vi "2DdblArrayTostrTable.vi"(7 "RowsAreStrings (f)":bool, 11 "dbl2DArray":dbl[][](array[numeric])) -> (3 "strTable":string[][](table))   [LabVIEW 2014, in "Framework.lvlib"]
uses:
  Framework.lvlib
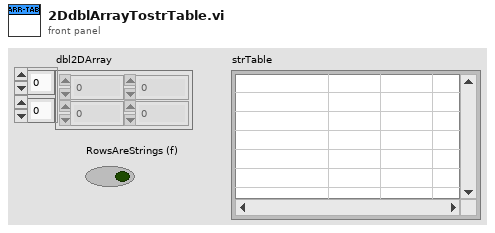
[diagram p1: front panel]
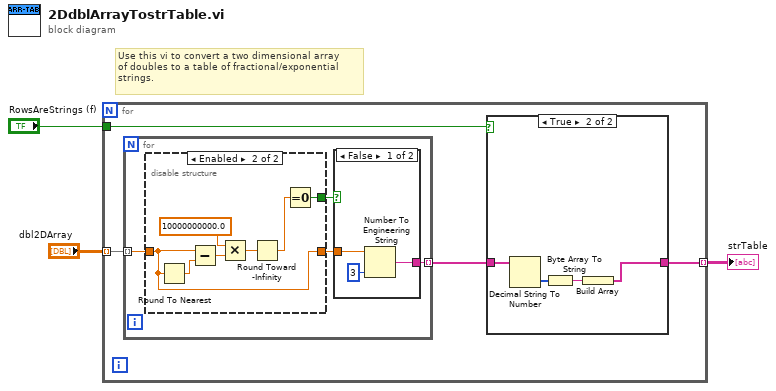
[diagram p0: block diagram]
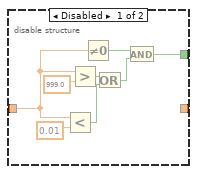
[diagram p3: hidden frame]
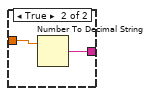
[diagram p4: hidden frame]
diagram:
  # "Use this vi to convert a two dimensional array \nof doubles to a table of fractional/exponential \nstrings."
  n1 = for {
    tunnel: [w4] -> w2 mode=indexing
    tunnel: "dbl2DArray" -> [w7] mode=indexing
    tunnel: "RowsAreStrings (f)" -> [w6]
    n2 = for {
      tunnel: [w16] -> w5 mode=indexing
      tunnel: w7 -> [w15] mode=indexing
      n3 = disable-structure shown="Enabled" {
        disable-tunnel: w15 -> [w18 w27]
        disable-tunnel: [w17 w26] -> w14
        disable-tunnel: [_ w27] -> w13
        frame Disabled {
          n4 = Less?(x=w18, y=0.01) -> (x < y?=w21:bool)
          n5 = Greater?(x=w18, y=999.0) -> (0:w22:bool)
          n6 = Not Equal To 0?(x=w18) -> (x != 0?=w20:bool)
          n7 = Or(x=w22, y=w21) -> (x .or. y?=w19:bool)
          n8 = And(x=w20, y=w19) -> (x .and. y?=w17:bool)
        }
        frame Enabled {
          n9 = Round To Nearest(number=w27) -> (nearest integer value=w31:dbl)
          n10 = Subtract(x=w27, y=w31) -> (x-y=w30:dbl)
          n11 = Multiply(x=10000000000.0, y=w30) -> (x*y=w28:dbl)
          n12 = Round Toward -Infinity(1:w28) -> (0:w25:dbl)
          n13 = Equal To 0?(x=w25) -> (x = 0?=w26:bool)
        }
      }
      n14 = case shown="False" w14 {
        tunnel: [w34 w36] -> w16
        tunnel: w13 -> [w33 w35]
        frame False {
          n15 = Number To Engineering String(2:i16 3 ("precision (6)"), 4:w33) -> (0:w34:string)  [unwired: 2 in]
        }
        frame True {
          n16 = Number To Decimal String(number=w35) -> (decimal integer string=w36:string)  [unwired: 1 in]
        }
      }
    }
    n17 = case shown="True" w6 {
      tunnel: w5 -> [w8 w12]
      tunnel: [w8 w9] -> w4
      frame False {
      }
      frame True {
        n18 = Decimal String To Number(string=w12) -> (number=w11:i32[])  [unwired: 2 in, 1 out]
        n19 = Byte Array To String(unsigned byte array=w11) -> (string=w10:string)
        n20 = Build Array(w10) -> (w9:string[])
      }
    }
  }
  "strTable" <- w2
